vi "Main.vi"(8 "error in (no error)":errorcluster, 11 "Module in":refnum<class "Module.lvclass">) -> (0 "error out":errorcluster, 3 "Module out":refnum<class "Module.lvclass">)   [LabVIEW 2021, in "Architecture.lvlib" / "Module.lvclass"]
uses:
  Module.lvclass
  Message/Message.lvclass
  Module.lvclass/Module.ctl
  Read user event.vi
  Read message queue.vi
  Message/Enqueue Multiple Messages.vi
  Message/Enqueue Single Message.vi
panel:
  in  "Stop Module":bool
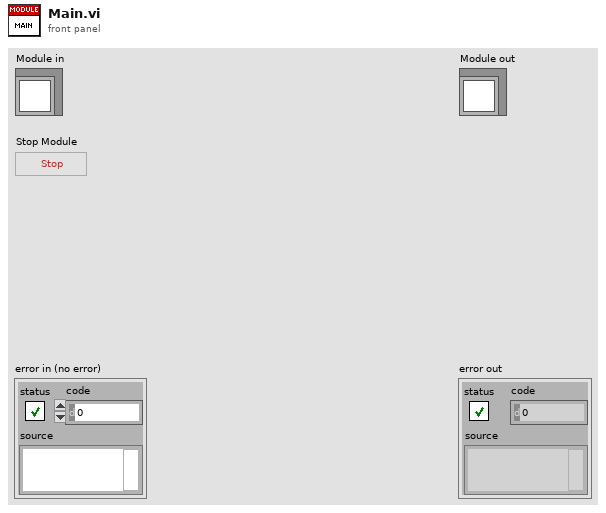
[diagram p1: front panel]
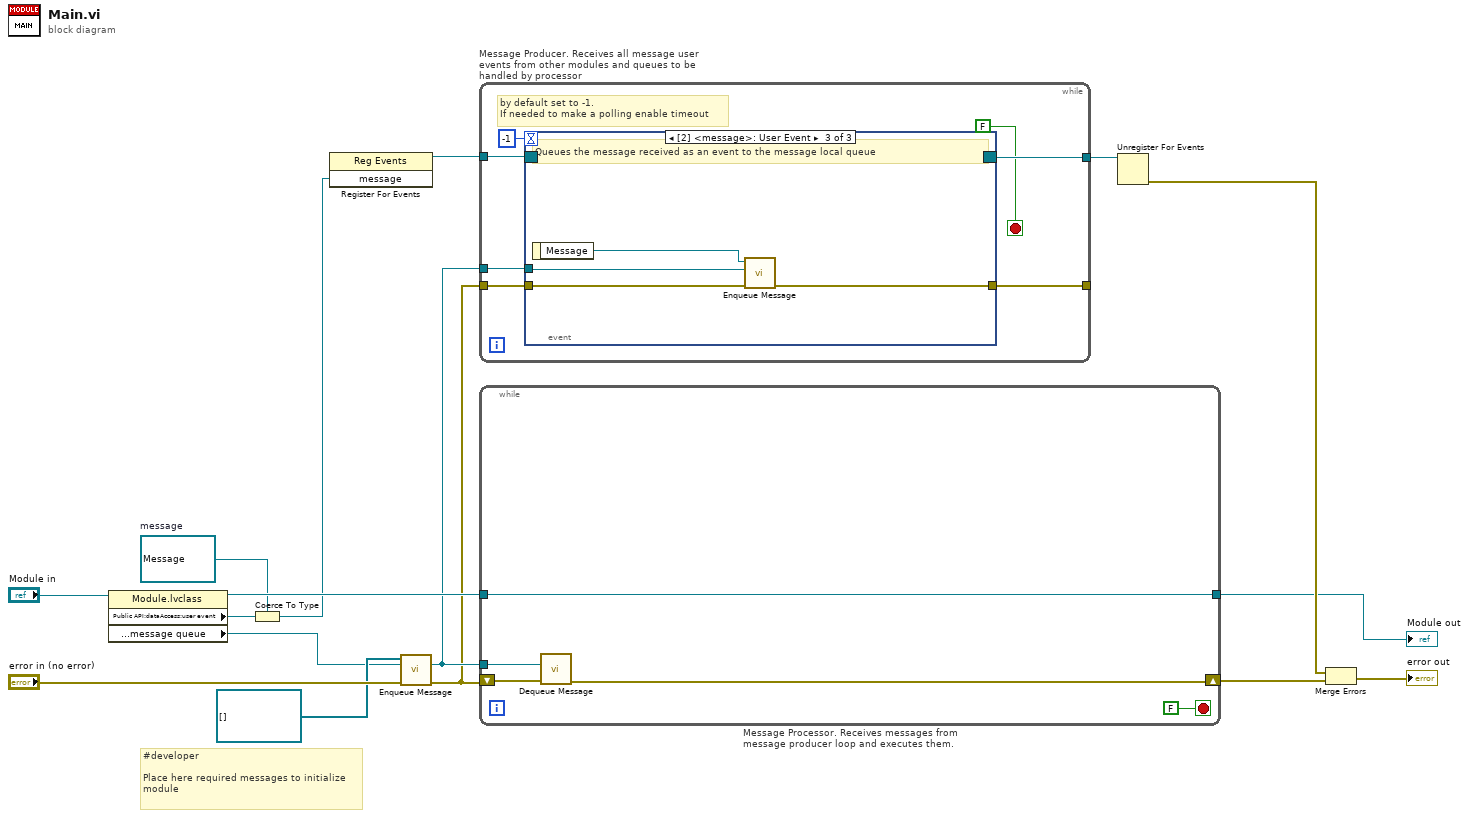
[diagram p0: block diagram]
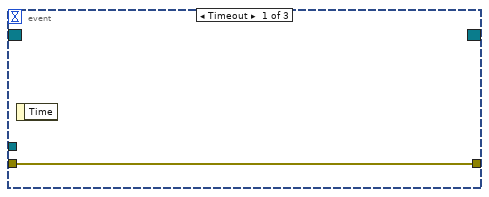
[diagram p2: hidden frame]
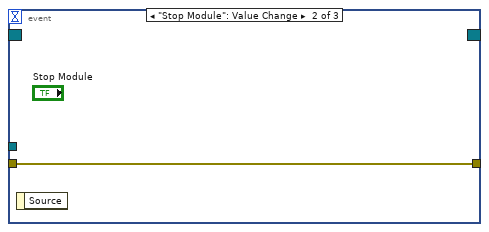
[diagram p3: hidden frame]
diagram:
  w2 = refnum<user-event> refnum  # message
  # "#developer\n\nPlace here required messages to initialize \nmodule"
  n1 = property class="Module.lvclass"(reference="Module in") -> (reference out=w7:refnum<class "Module.lvclass">, "Public API:dataAccess:user event"=w11:refnum<user-event>, "Public API:dataAccess:message queue"=w12:refnum<queue>)  [unwired: 1 in, 1 out]
  n2 = Coerce To Type(0:w11, 1:w2) -> (2:w3:refnum<user-event>)
  n3 = register-events(w3) -> (reference out=w4:refnum<event-registration>)  [unwired: 2 in, 1 out]
  n4 = call-poly "Enqueue Message.vi"("error in (no error)"="error in (no error)", "queue in"=w12, "Message in"=refnum<class "Message.lvclass">[] []) -> ("error out"=w5:errorcluster, "queue out"=w6:refnum<queue>)  [unwired: 7 in]
  n5 = while "Message Producer. Receives all message user events from other modules and queues to be handled by processor" {
    tunnel: w4 -> [w23]
    tunnel: [w22] -> w10
    tunnel: w6 -> [w21]
    tunnel: w5 -> [w20]
    tunnel: [w18] -> _
    stop <- FALSE stop-if-true
    # "by default set to -1. \nIf needed to make a polling enable timeout"
    n6 = event shown="[2] <message>: User Event" {
      selector: w23 -> [_ _ _]
      dyn-events: [_ _ _] -> w22
      timeout: -1 -> [_ _ _]
      tunnel: w21 -> [_ _ w27]
      tunnel: w20 -> [w24 w25 w29]
      tunnel: [w24 w25 w28] -> w18
      event Timeout {
        n7 = event-data() -> ()  [unwired: 1 in, 1 out]
      }
      event "Stop Module": Value Change {
        n8 = event-data() -> ()  [unwired: 1 in, 1 out]
      }
      event User Event {
        # "Queues the message received as an event to the message local queue"
        n9 = event-data() -> ("Message"=w26:refnum<class "Message.lvclass">)  [unwired: 1 in]
        n10 = call-poly "Enqueue Message.vi"("error in (no error)"=w29, "queue in"=w27, "Message in"=w26) -> ("error out"=w28:errorcluster)  [unwired: 7 in, 1 out]
      }
    }
  }
  n11 = while "Message Processor. Receives messages from message producer loop and executes them." {
    tunnel: w6 -> [w34]
    shift-right: [w32] -> w16
    shift-left: w5 -> [w33]
    tunnel: w7 -> [w30]
    tunnel: [w30] -> w1
    stop <- FALSE stop-if-true
    n12 = call "Dequeue Message.vi"("error in (no error)"=w33, "queue in"=w34) -> ("error out"=w32:errorcluster)  [unwired: 7 in, 2 out]
  }
  "Module out" <- w1
  n13 = Unregister For Events(event registration refnum=w10) -> (error out=w8:errorcluster)  [unwired: 1 in]
  n14 = Merge Errors(w8, w16) -> (→"error out":errorcluster)
